vi "ConvertToU8matrix.vi"(11 "Image In":T1) -> (1 "Intensity Graph":u8[][](graph), 3 "Image out":T1)   [LabVIEW 2019]
uses:
  <vilib>/picture/picture.llb/imagedata.ctl
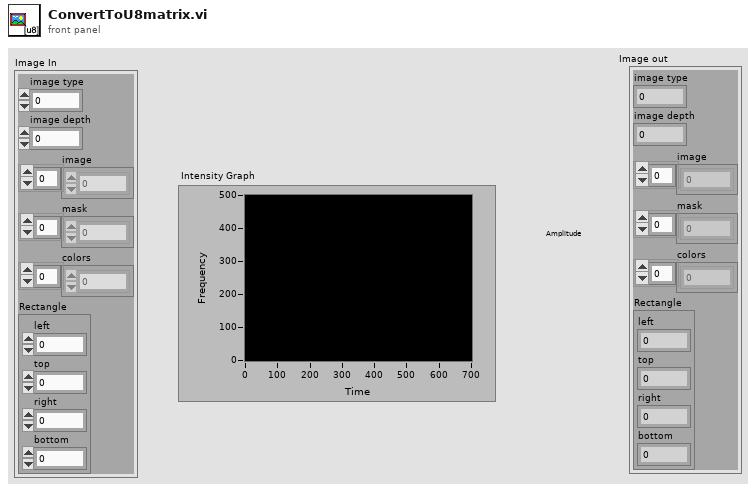
[diagram p1: front panel]
types:
  T1 = typedef "imagedata.ctl" = cluster{"image type":i32, "image depth":i32, "image":u8[], "mask":u8[], "colors":u32[], "Rectangle":cluster{"left":i16, "top":i16, "right":i16, "bottom":i16}}
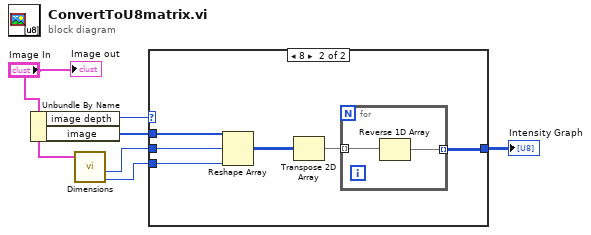
[diagram p0: block diagram]
diagram:
  n1 = Unbundle By Name("Image In") -> ("image depth"=w4:i32, "image"=w5:u8[])
  n2 = call "Dimensions.vi"("Image In"="Image In") -> ("width"=w1:i32, "height"=w2:i32)  [unwired: 8 in, 1 out]
  n3 = case shown="8" w4 {
    tunnel: w5 -> [_ w10]
    tunnel: w2 -> [_ w12]
    tunnel: w1 -> [_ w11]
    tunnel: [_ w7] -> w6
    frame 0, Default {
    }
    frame 8 {
      n4 = Reshape Array(w10, w12, w11) -> (w9:u8[][])
      n5 = Transpose 2D Array(2D array=w9) -> (transposed array=w8:u8[][])
      n6 = for {
        tunnel: w8 -> [w14] mode=indexing
        tunnel: [w13] -> w7 mode=indexing
        n7 = Reverse 1D Array(array=w14) -> (reversed array=w13:u8[])
      }
    }
  }
  "Intensity Graph" <- w6
  "Image out" <- "Image In"
